vi "AddTag.vi"(8 "error in (no error)":errorcluster, 9 "TupeTerminode":enum16{"Tag", "Child"}(ring), 10 "CreateNameTag":string, 11 "ClassDataTree in":refnum<class "ClassDataTree.lvclass">) -> (0 "error out":errorcluster, 3 "ClassDataTree out":refnum<class "ClassDataTree.lvclass">)   [LabVIEW 2010, in "ClassDataTree.lvclass"]
uses:
  ClassDataTree.lvclass
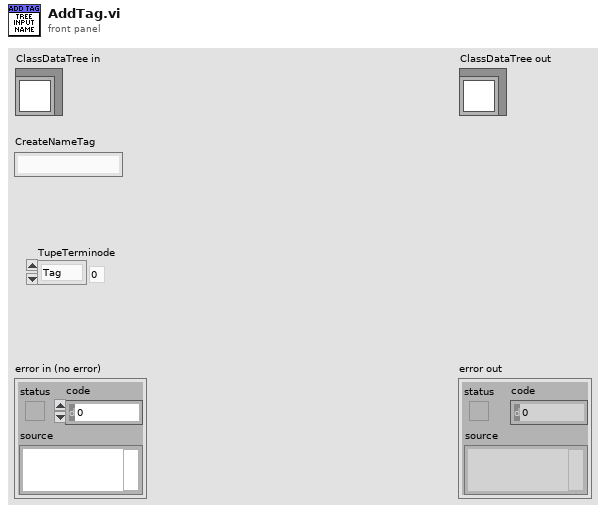
[diagram p1: front panel]
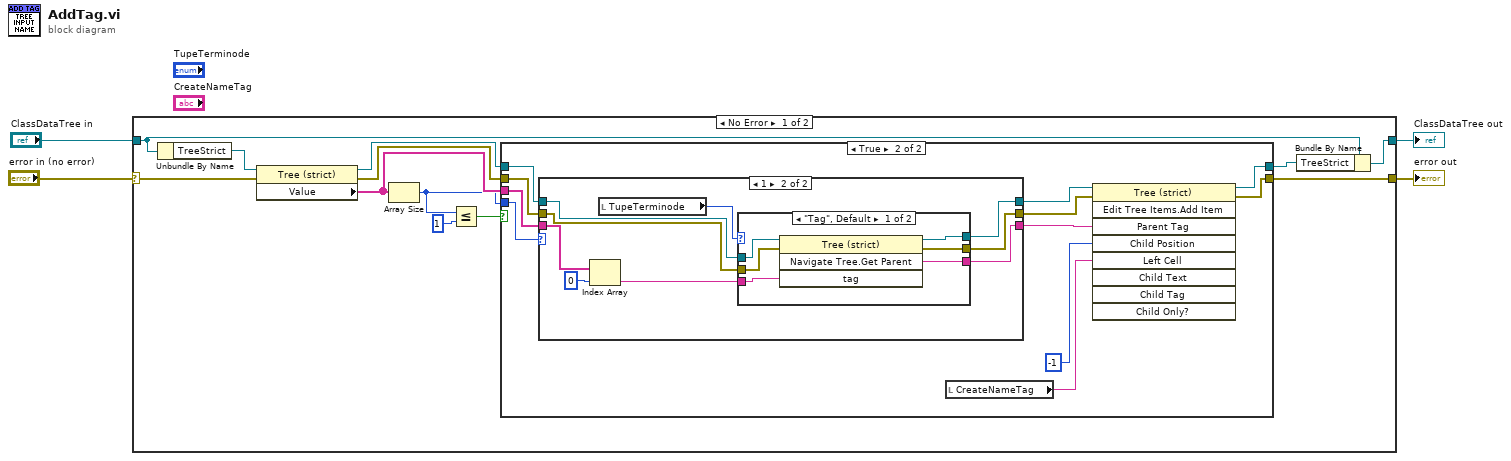
[diagram p0: block diagram]
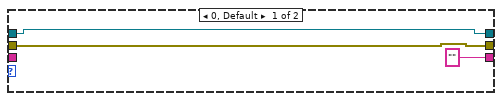
[diagram p3: hidden frame]
diagram:
  n1 = case shown="No Error" "error in (no error)" {
    selector: "error in (no error)" -> [w13 w52]
    tunnel: [w11 w52] -> w3
    tunnel: [w5 w51] -> w1
    tunnel: "ClassDataTree in" -> [w7 w51]
    frame No Error {
      n2 = Unbundle By Name(w7) -> ("TreeStrict"=w16:refnum<vi>)
      n3 = property class="Tree (strict)"(reference=w16, error in=w13) -> (reference out=w14:refnum<vi>, error out=w12:errorcluster, "Value"=w15:string[])
      n4 = Array Size(array=w15) -> (size(s)=w10:i32)
      n5 = Less Or Equal?(x=w10, y=1) -> (x <= y?=w8:bool)
      n6 = case shown="True" w8 {
        tunnel: w15 -> [_ w29]
        tunnel: w14 -> [w18 w22]
        tunnel: w12 -> [w17 w21]
        tunnel: [w17 w28] -> w11
        tunnel: w10 -> [_ w25]
        tunnel: [w18 w24] -> w6
        frame False {
        }
        frame True {
          n7 = case shown="1" w25 {
            tunnel: w29 -> [_ w41]
            tunnel: ["" w34] -> w23
            tunnel: w22 -> [w31 w39]
            tunnel: w21 -> [w30 w38]
            tunnel: [w31 w37] -> w20
            tunnel: [w30 w36] -> w19
            frame 0, Default {
            }
            frame 1 {
              n8 = Index Array(array=w41, index=0) -> (element=w35:string)
              n9 = local read "TupeTerminode"() -> (w33:enum16{"Tag", "Child"})
              n10 = case shown="\"Tag\", Default" w33 {
                tunnel: w39 -> [w47 w50]
                tunnel: w38 -> [w46 w49]
                tunnel: [w45 w50] -> w37
                tunnel: [w44 w49] -> w36
                tunnel: w35 -> [w43 w48]
                tunnel: [w42 w48] -> w34
                frame "Tag", Default {
                  n11 = invoke class="Tree (strict)" method="Navigate Tree.Get Parent"(reference=w47, error in=w46, "tag"=w43) -> (reference out=w45:refnum<vi>, error out=w44:errorcluster, "Navigate Tree:Get Parent"=w42:string)  [unwired: 1 in, 1 out]
                }
                frame "Child" {
                }
              }
            }
          }
          n12 = local read "CreateNameTag"() -> (w26:string)
          n13 = invoke class="Tree (strict)" method="Edit Tree Items.Add Item"(reference=w20, error in=w19, "Parent Tag"=w23, "Child Position"=-1, "Left Cell"=w26) -> (reference out=w24:refnum<vi>, error out=w28:errorcluster)  [unwired: 4 in, 7 out]
        }
      }
      n14 = Bundle By Name(cluster=w7, "TreeStrict"=w6) -> (w5:refnum<class "ClassDataTree.lvclass">)
    }
    frame Error {
    }
  }
  "error out" <- w3
  "ClassDataTree out" <- w1
